vi "Trigger Manager Subpanel Manager Connect Event.vi"(8 "error in (no error)":errorcluster, 11 "CIF_Manager_UI in":refnum<class "CIF_Manager_UI.lvclass">) -> (0 "error out":errorcluster)   [LabVIEW 2021, in "CIF_Manager_UI.lvclass"]
uses:
  CIF_Manager_UI.lvclass
  C:/Program Files/National Instruments/LabVIEW 2021/vi.lib/CIF Foundation/CIF Core/CIFUI/CIF_UI.lvclass
  CIF_Manager_UI.lvclass/CIF_Manager_UI.ctl
  <vilib>/CIF Foundation/CIF Core/CIFUI/CIF_UI.lvclass/CIF_UI.ctl
  <vilib>/CIF Foundation/CIF Core/CIFUI/Accessors/Read Manager gRPC ID.vi
  <vilib>/CIF Foundation/CIF Core/CIFUI/Accessors/Read IP Address.vi
  <vilib>/CIF Foundation/CIF Core/CIFUI/Accessors/Read Connected.vi
  <vilib>/gRPC/LabVIEW gRPC Library/Shared/grpcId.ctl
  <vilib>/gRPC/LabVIEW gRPC Library/grpc-lvsupport-release.lvlib
  CIFPluginManager/typedef/New Connection Event Data.ctl
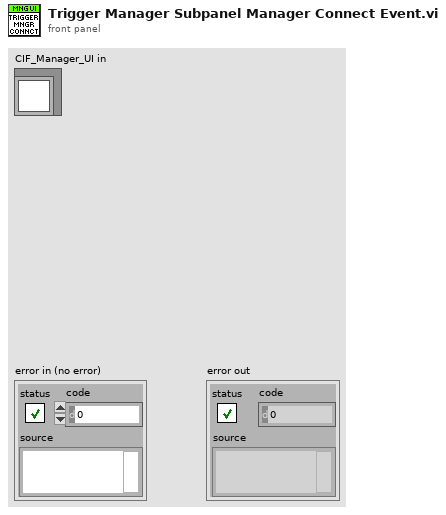
[diagram p1: front panel]
types:
  T1 = typedef "CIF_Manager_UI.lvclass/New Connection Event Data.ctl" = cluster{"Manager gRPC ID":T2, "IP Address":string, "Connected":bool}
  T2 = typedef "grpc-lvsupport-release.lvlib/grpcId.ctl" = u64
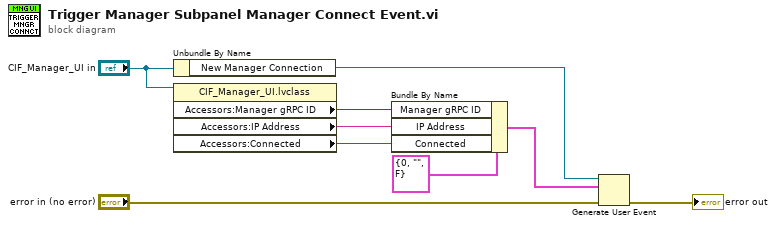
[diagram p0: block diagram]
diagram:
  n1 = Unbundle By Name("CIF_Manager_UI in") -> ("New Manager Connection"=w1:refnum<user-event>)
  n2 = property class="CIF_Manager_UI.lvclass"(reference="CIF_Manager_UI in") -> ("Accessors:Manager gRPC ID"=w6:T2, "Accessors:IP Address"=w4:string, "Accessors:Connected"=w3:bool)  [unwired: 1 in, 2 out]
  n3 = Bundle By Name(cluster=T1 {"Manager gRPC ID"=0, "IP Address"="", "Connected"=FALSE} ("gRPC Connection Data"), "Manager gRPC ID"=w6, "IP Address"=w4, "Connected"=w3) -> (w5:T1)
  n4 = Generate User Event(user event=w1, event data cluster=w5, error in="error in (no error)") -> (error out=→"error out":errorcluster)  [unwired: 1 in, 1 out]
